vi "FABR-Compute Thresholds.vi"(0 "Analysis in":T2, 13 "Threshold Estimation":T3) -> (4 "Analysis out":T2)   [LabVIEW 2020]
uses:
  Threshold Estimation VIs/ABR3-Threshold Estimation Parameters.ctl
  Typedefs/FABR-Analysis State.ctl
  Threshold Estimation VIs/ABR3-Threshold Estimation Result.ctl
panel:
  in  "Result":T1
  # "Freq X Level X Time"
  # "Freq X Level X Time"
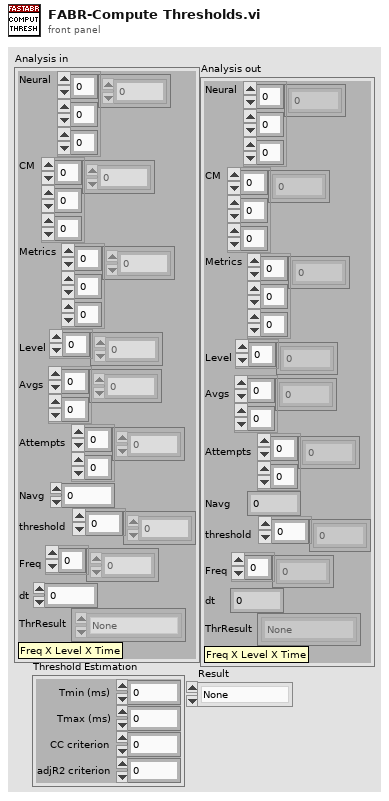
[diagram p1: front panel]
types:
  T1 = typedef "ABR3-Threshold Estimation Result.ctl" = enum16{"None", "Power", "Sigmoid", "Power (noisy)", "Suprathreshold", "Invalid"}
  T2 = typedef "FABR-Analysis State.ctl" = cluster{"Neural":dbl[][][], "CM":dbl[][][], "Metrics":dbl[][][], "Level":dbl[], "Avgs":i32[][], "Attempts":i32[][], "Navg":i32, "threshold":dbl[], "Freq":dbl[], "dt":dbl, "ThrResult":T1[]}
  T3 = typedef "ABR3-Threshold Estimation Parameters.ctl" = cluster{"Tmin (ms)":dbl, "Tmax (ms)":dbl, "CC criterion":dbl, "adjR2 criterion":dbl}
  T4 = typedef "ABR3-Threshold Estimation Work.ctl" = cluster{"Threshold":dbl, "Criterion":dbl, "graphs":cluster{"X":dbl[], "Y":dbl[]}[], "Power2":string, "Sigmoid":string, "Result":T1}
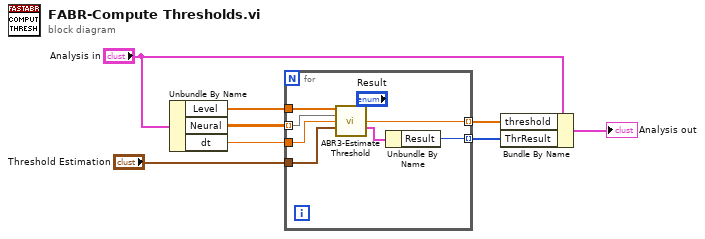
[diagram p0: block diagram]
diagram:
  n1 = Unbundle By Name("Analysis in") -> ("Level"=w8:dbl[], "Neural"=w7:dbl[][][], "dt"=w2:dbl)
  n2 = for {
    tunnel: w8 -> [w15]
    tunnel: w7 -> [w14] mode=indexing
    tunnel: "Threshold Estimation" -> [w13]
    tunnel: [w12] -> w4 mode=indexing
    tunnel: w2 -> [w11]
    tunnel: [w9] -> w1 mode=indexing
    n3 = call "ABR3-Estimate Threshold.vi"("Level (in)"=w15, "Neural"=w14, "dt (us)"=w11, "Threshold Estimation"=w13) -> ("Threshold"=w12:dbl, "Work"=w10:T4)  [unwired: 9 in, 1 out]
    n4 = Unbundle By Name(w10) -> ("Result"=w9:T1)
  }
  n5 = Bundle By Name(cluster="Analysis in", "threshold"=w4, "ThrResult"=w1) -> (→"Analysis out":T2)
